vi "Get Recursive Owned VIs List.vi"(0 "Parent[]":refnum<vi>[](array[refnum])) -> (4 "Children[]":refnum<vi>[](array[refnum]))   [LabVIEW 2018, in "Springboard TLB`.lvlib"]
uses:
  Springboard TLB`.lvlib
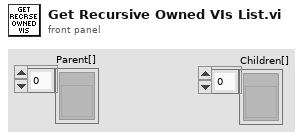
[diagram p1: front panel]
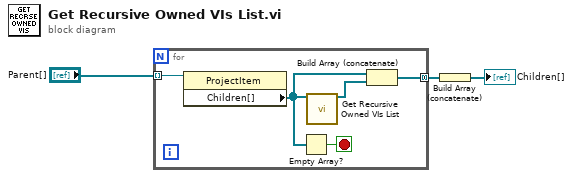
[diagram p0: block diagram]
diagram:
  n1 = for {
    tunnel: "Parent[]" -> [w8] mode=indexing
    tunnel: [w5] -> w3 mode=concatenating
    stop <- w7 stop-if-true
    n2 = property class="ProjectItem"(reference=w8) -> ("Children[]"=w6:refnum<vi>[])  [unwired: 1 in, 2 out]
    n3 = Empty Array?(array=w6) -> (empty?=w7:bool)
    n4 = call "Get Recursive Owned VIs List.vi"("Parent[]"=w6) -> ("Children[]"=w4:refnum<vi>[])  [unwired: 14 in]
    n5 = Build Array (concatenate)(w6, w4) -> (w5:refnum<vi>[])
  }
  n6 = Build Array (concatenate)(w3) -> (→"Children[]":refnum<vi>[])
